vi "Read local path.vi"(8 "error in":errorcluster, 11 "Shared Library Module editor node in":refnum<class "Shared Library Module editor node.lvclass">) -> (0 "error out":errorcluster, 2 "local path":path, 3 "Shared Library Module editor node out":refnum<class "Shared Library Module editor node.lvclass">)   [LabVIEW 2013, in "Shared Library Module editor node.lvclass"]
uses:
  Shared Library Module editor node.lvclass
  <vilib>/NI/Tag Bus Data Framework/Configuration Editor/Classes/Module editor node/module editor node.lvclass
  <vilib>/NI/Configuration Framework/serializable configuration/NISE_CEF_serializable configuration.lvclass
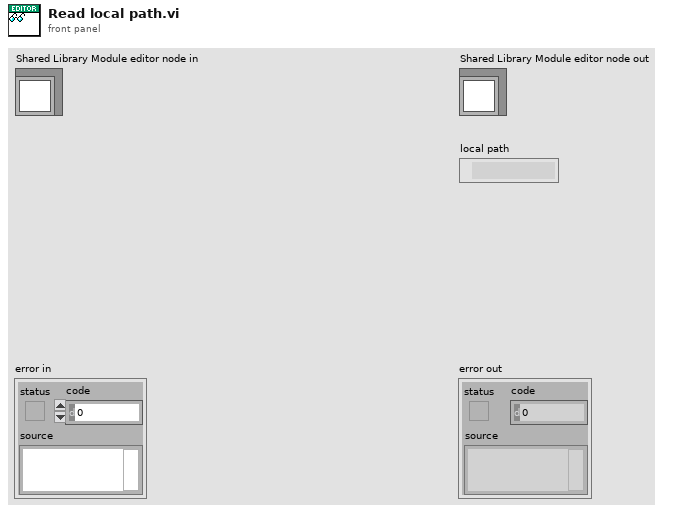
[diagram p1: front panel]
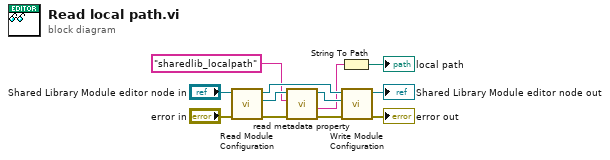
[diagram p0: block diagram]
diagram:
  n1 = call <vilib>:"Read Module Configuration.vi"("error in"="error in", "Module Editor Node in"="Shared Library Module editor node in") -> ("error out"=w10:errorcluster, "module configuration"=w11:refnum<class "TBM module configuration.lvclass">, "Module Editor Node out"=w12:refnum<class "Shared Library Module editor node.lvclass">)  [unwired: 7 in]
  n2 = call <vilib>:"read metadata property.vi"("error in"=w10, "key"="sharedlib_localpath", "configuration in"=w11) -> ("error out"=w8:errorcluster, "value"=w2:string, "configuration out"=w9:refnum<class "TBM module configuration.lvclass">)  [unwired: 5 in, 1 out]
  n3 = String To Path(string=w2) -> (path=→"local path":path)
  n4 = call <vilib>:"Write Module Configuration.vi"("error in"=w8, "module configuration"=w9, "Module Editor Node in"=w12) -> ("error out"=→"error out":errorcluster, "Module Editor Node out"=→"Shared Library Module editor node out":refnum<class "Shared Library Module editor node.lvclass">)  [unwired: 7 in]
